vi "Unpickle.vi"(0 "pickle":string, 11 "error in (no error)":errorcluster) -> (4 "variant":variant, 15 "error out":errorcluster)   [LabVIEW 2015, in "LV Exceptions v1.lvlib"]
doc: "This function is compimentary to 'Pickle'."
uses:
  LV Exceptions v1.lvlib
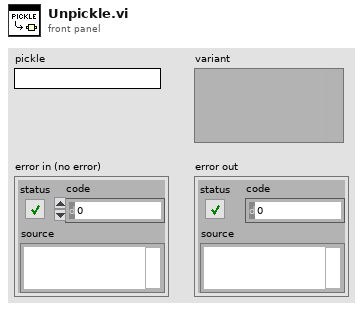
[diagram p1: front panel]
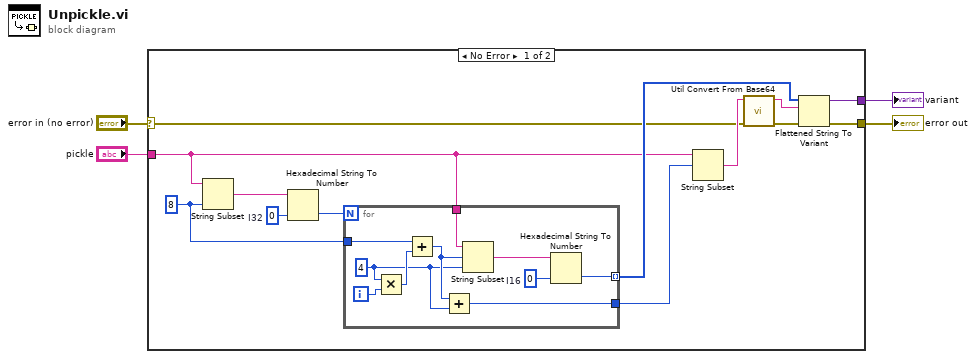
[diagram p0: block diagram]
diagram:
  n1 = case shown="No Error" "error in (no error)" {
    selector: "error in (no error)" -> [w5 w28]
    tunnel: [w9 _] -> w4
    tunnel: "pickle" -> [w8 _]
    tunnel: [w6 w28] -> w2
    frame No Error {
      w16 = 0  # I32
      w14 = 8 ("length (rest)")
      n2 = String Subset(string=w8, length (rest)=w14) -> (substring=w15:string)  [unwired: 1 in]
      n3 = Hexadecimal String To Number(string=w15, default (0uL)=w16) -> (number=w13:i32)  [unwired: 1 in, 1 out]
      n4 = for {
        N: w13 -> [_]
        tunnel: w14 -> [w25]
        tunnel: [w24] -> w10 mode=indexing
        tunnel: [w19] -> w12
        tunnel: w8 -> [w18]
        i -> [w27]
        w22 = i16 0  # I16
        w20 = 4
        n5 = Multiply(x=w20, y=w27) -> (x*y=w26:i32)
        n6 = Add(x=w25, y=w26) -> (x+y=w21:i32)
        n7 = Add(x=w21, y=w20) -> (x+y=w19:i32)
        n8 = String Subset(string=w18, offset (0)=w21, length (rest)=w20) -> (substring=w23:string)
        n9 = Hexadecimal String To Number(string=w23, default (0uL)=w22) -> (number=w24:i16)  [unwired: 1 in, 1 out]
      }
      n10 = String Subset(string=w8, offset (0)=w12) -> (substring=w11:string)  [unwired: 1 in]
      n11 = call "Util Convert From Base64.vi"("error in (no error)"=w5, "Base64 String"=w11) -> ("error out"=w7:errorcluster, "String"=w17:string)  [unwired: 8 in]
      n12 = Flattened String To Variant(4:w7, 6:w17, 7:w10) -> (0:w6:errorcluster, 3:w9:variant)
    }
    frame Error {
    }
  }
  "error out" <- w2
  "variant" <- w4
